vi "SetHeadEnableStatus_GIS Printer.vi"(7 "ForceEvent":bool, 8 "error in (no error)":errorcluster, 9 "Value":string, 10 "Command":string, 11 "GIS Printer In":refnum<class "GIS Printer.lvclass">) -> (0 "error out":errorcluster, 3 "GIS Printer Out":refnum<class "GIS Printer.lvclass">)   [LabVIEW 2022 SP3, in "GIS Printer.lvclass"]
uses:
  GIS Printer.lvclass
  GIS Printer.lvclass/GIS Printer.ctl
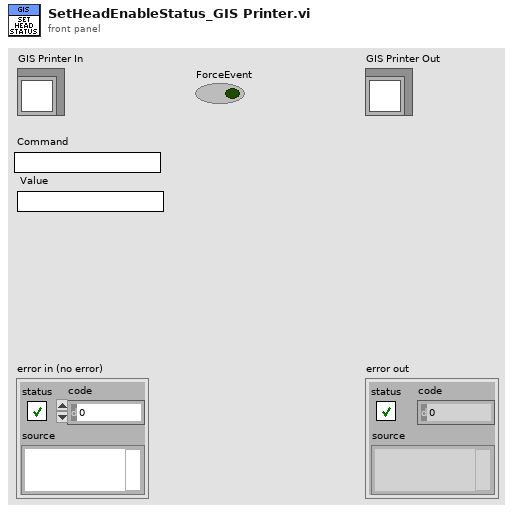
[diagram p1: front panel]
types:
  T1 = typedef "GIS Printer.lvclass/Private Data.ctl" = cluster{"UserEvents":T2, "All Dependencies":cluster{"Class References":refnum<class>[], "Class Names":string[]}, "PrinterConiguration":T3, "Status":T4, "GISHeadStatus":T5[], "HeadStatus":T6}
  T2 = typedef "GIS Printer.lvclass/UserEvents.ctl" = cluster{"API Incoming Event":refnum<user-event>, "API Executed Event":refnum<user-event>, "API Return Event":refnum<user-event>, "Status Changed Event":refnum<user-event>, "Abort":refnum<user-event>, "stop process":refnum<user-event>, "GISPollStatus":refnum<user-event>, "GISHeadStatus":refnum<user-event>, "Error Event":refnum<user-event>}
  T3 = typedef "GIS Printer.lvclass/PrinterConfiguration--Cluster.ctl" = cluster{"IPAddress":string, "Move Stage on RTP Command?":bool, "Stage Move Position":string, "PH1-Prime Path":path, "PH2-Prime Path":path, "PH3-Prime Path":path, "PH4-Prime Path":path, "PH5-Prime Path":path, "PH6-Prime Path":path, "PrintScriptsFolder":path, "PurgeScriptsFolder":path, "StageScriptsFolder":path, "PH1-HeatOn Path":path, "PH2-HeatOn Path":path, "PH3-HeatOn Path":path, "PH4-HeatOn Path":path, "PH5-HeatOn Path":path, "PH6-HeatOn Path":path, "PH1-HeatOff Path":path, "PH2-HeatOff Path":path, "PH3-HeatOff Path":path, "PH4-HeatOff Path":path, "PH5-HeatOff Path":path, "PH6-HeatOff Path":path}
  T4 = typedef "GIS Printer.lvclass/Status Cluster.ctl" = cluster{"Command Status":variant, "TCP Commands & Responses":string[][], "Printer Busy?":bool}
  T5 = typedef "GIS Status--Cluster.ctl" = cluster{"HeadEnabled":bool, "SpitEnabled":bool, "HeaterEnabled":bool, "TargetTemperature":dbl, "CurrentTemperature":dbl}
  T6 = typedef "HeadEnableStatus--cluster.ctl" = cluster{"PH1_Enable":bool, "PH2_Enable":bool, "PH3_Enable":bool, "PH4_Enable":bool, "PH5_Enable":bool, "PH6_Enable":bool}
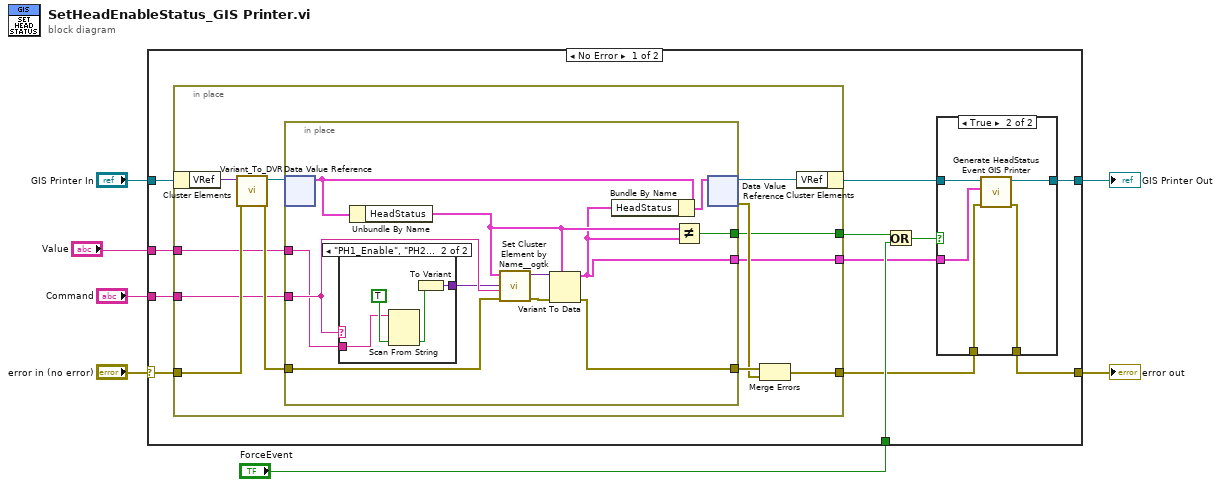
[diagram p0: block diagram]
diagram:
  n1 = case shown="No Error" "error in (no error)" {
    selector: "error in (no error)" -> [w18 w56]
    tunnel: [w8 w56] -> w6
    tunnel: [w11 w55] -> w4
    tunnel: "GIS Printer In" -> [w19 w55]
    tunnel: "Command" -> [w17 _]
    tunnel: "Value" -> [w16 _]
    tunnel: "ForceEvent" -> [w14 _]
    frame No Error {
      n2 = in-place {
        in-place-border: w18 -> [w36]
        in-place-border: [w32] -> w9
        in-place-border: w17 -> [w30]
        in-place-border: w16 -> [w29]
        in-place-border: [w28] -> w15
        in-place-border: [w27] -> w10
        n3 = in-place-cluster #1(w19) -> ("VRef"=w38:variant)
        n4 = call "Variant_To_DVR.vi"("error in (no error)"=w36, "Variant"=w38) -> ("error out"=w35:errorcluster, "DVR"=w37:refnum<data-value>)  [unwired: 8 in]
        n5 = in-place {
          in-place-border: w35 -> [w47]
          in-place-border: [w45] -> w34
          in-place-border: w30 -> [w44]
          in-place-border: w29 -> [w43]
          in-place-border: [w40] -> w28
          in-place-border: [w39] -> w27
          n6 = in-place-dvr #2(w37) -> (w50:T1)  [unwired: 1 out]
          n7 = case shown="\"PH1_Enable\", \"PH2_Enable\", \"PH3_Enable\", \"PH4_Enable\", \"PH5_Enable\", \"PH6_Enable\"" w44 {
            tunnel: w43 -> [_ w53]
            tunnel: [_ w51] -> w42
            frame "False", Default {
            }
            frame "PH1_Enable", "PH2_Enable", "PH3_Enable", "PH4_Enable", "PH5_Enable", "PH6_Enable" {
              n8 = Scan From String(input string=w53, default 1=TRUE) -> (output 1=w52:bool)  [unwired: 3 in, 3 out]
              n9 = To Variant(anything=w52) -> (Variant=w51:variant)
            }
          }
          n10 = Unbundle By Name(w50) -> ("HeadStatus"=w41:T6)
          n11 = call <userlib>:"Set Cluster Element by Name__ogtk.vi"("error in (no error)"=w47, "Element Name (\"\": New Element Data Name)"=w44, "New Element Value"=w42, "Cluster"=w41) -> ("error out"=w46:errorcluster, "VCluster out"=w48:variant)  [unwired: 5 in, 1 out]
          n12 = Variant To Data(error in=w46, type=w41, Variant=w48) -> (data=w39:T6, error out=w45:errorcluster)
          n13 = Bundle By Name(cluster=w50, "HeadStatus"=w39) -> (w49:T1)
          n14 = Not Equal?(x=w41, y=w39) -> (x != y?=w40:bool)
          n15 = in-place-dvr #2(w49) -> (w31:refnum<data-value>, w33:errorcluster)
        }
        n16 = Merge Errors(w34, w33) -> (w32:errorcluster)
        n17 = in-place-cluster #1("VRef"=w31) -> (w12:refnum<class "GIS Printer.lvclass">)
      }
      n18 = Or(x=w15, y=w14) -> (x .or. y?=w13:bool)
      n19 = case shown="True" w13 {
        tunnel: w12 -> [w21 w25]
        tunnel: [w21 w24] -> w11
        tunnel: w9 -> [w20 w23]
        tunnel: [w20 w22] -> w8
        tunnel: w10 -> [_ w26]
        frame False {
        }
        frame True {
          n20 = call "Generate HeadStatus Event GIS Printer.vi"("error in (no error)"=w23, "HeadStatus"=w26, "GIS Printer in"=w25) -> ("error out"=w22:errorcluster, "GIS Printer out"=w24:refnum<class "GIS Printer.lvclass">)  [unwired: 7 in]
        }
      }
    }
    frame Error {
    }
  }
  "error out" <- w6
  "GIS Printer Out" <- w4
